vi "DataViewer_Optics.vi"() -> ()   [LabVIEW 2019]
uses:
  <vilib>/Utility/file.llb/Read Delimited Spreadsheet (DBL).vi
panel:
  in  "Tab Control":T1(tab)
  out "Spectrum":cluster{dbl[], "all rows":dbl[]}(graph)
  in  "Spectrum File":path
  in  "Calibration File":path
  in  "Spectrum":bool
  in  "Mask A":path
  out "Mask A Transmission":dbl[][](graph)
  in  "Transmission":bool
  out "Mask B Transmission":dbl[][](graph)
  in  "Mask B":path
  in  "Pixel to Plot":dbl
  in  "Transmission_Px":bool
  in  "Mask A":path
  in  "Mask B":path
  out "Mask A":dbl[](graph)
  out "Mask B":dbl[](graph)
  in  "Pixel":dbl
  in  "Phase":bool
  in  "Directory":path
  out "SLM Phase Mask A":cluster{"all rows":dbl[], "all rows":dbl[]}(graph)
  out "SLM Phase Mask B":cluster{"all rows":dbl[], "all rows":dbl[]}(graph)
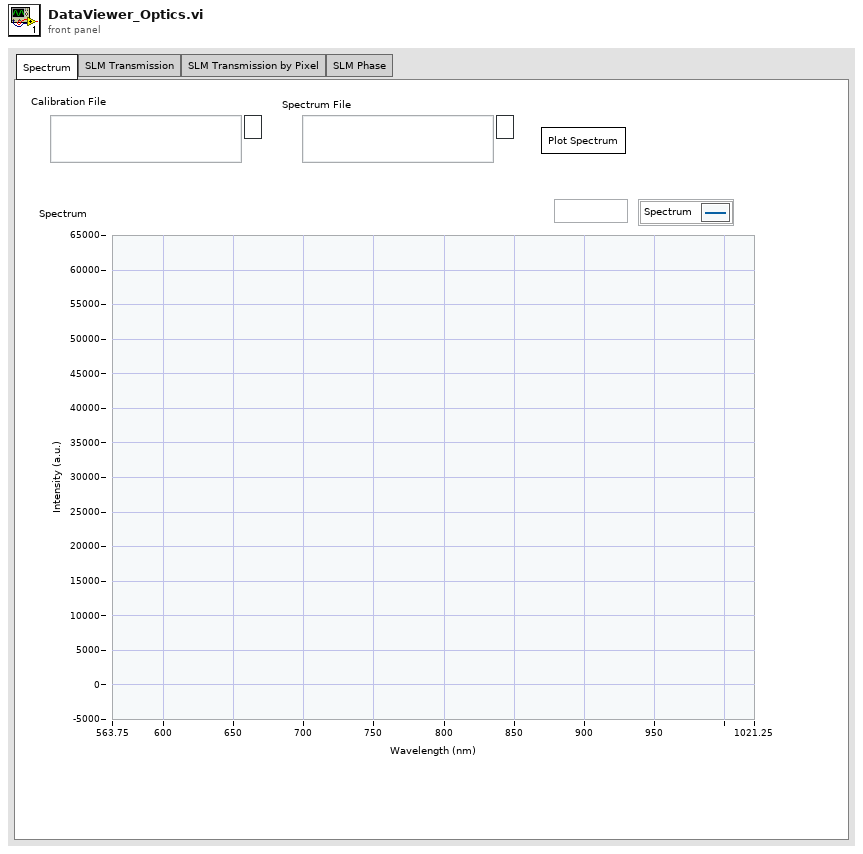
[diagram p1: front panel]
types:
  T1 = enum32{"Spectrum", "SLM Transmission", "SLM Transmission by Pixel", "SLM Phase"}
  T2 = enum32{"Invalid", "Standard", "Closed", "Hidden", "Minimized", "Maximized"}
  T3 = enum32{"invalid app kind", "Development System", "Run Time System", "Student Edition", "Embedded LabVIEW", "Evaluation", "Custom"}
  T4 = cluster{"Core":cluster{"Current VI Reference":refnum<vi>, "Close Panel on Exit?":bool}, "Your Boolean data":bool, "Your string data":string}
  T5 = cluster{"Current VI Reference":refnum<vi>, "Close Panel on Exit?":bool}
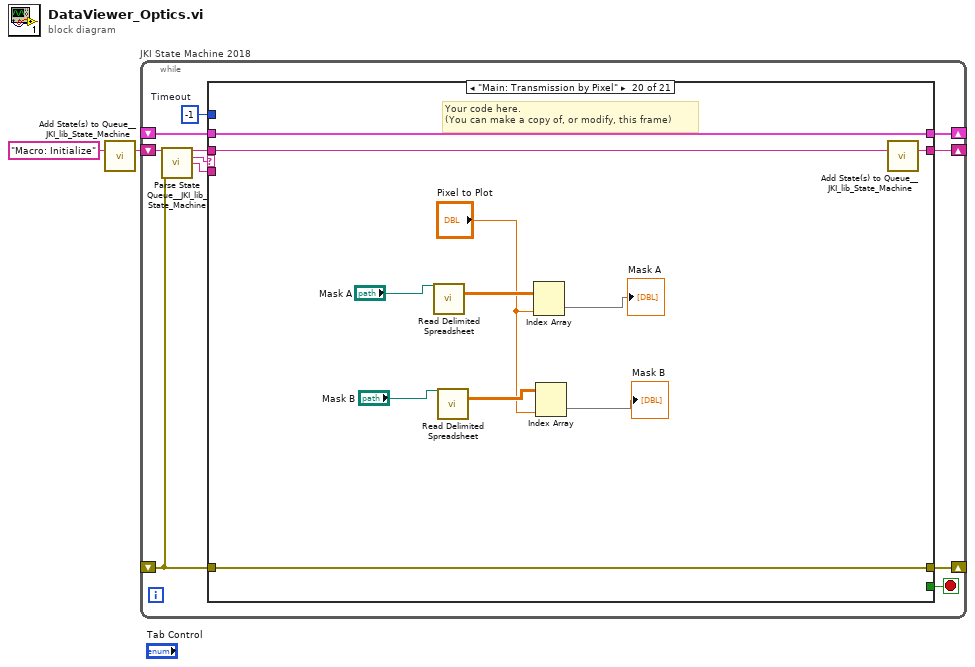
[diagram p0: block diagram]
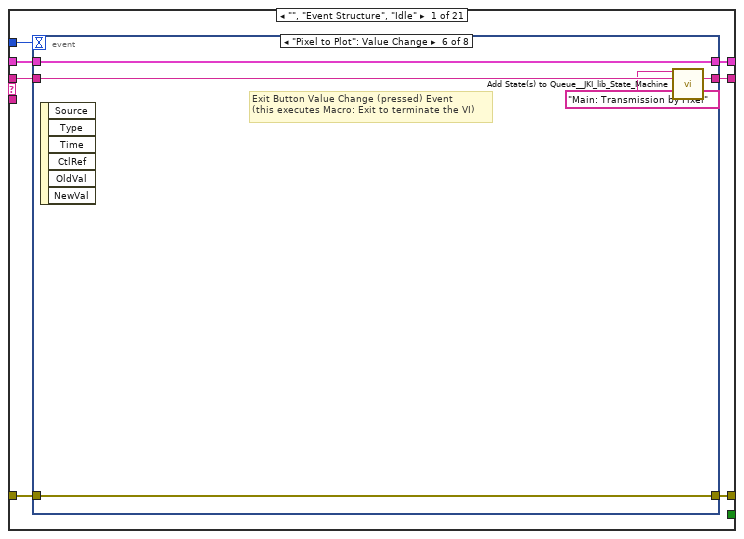
[diagram p2: hidden frame]
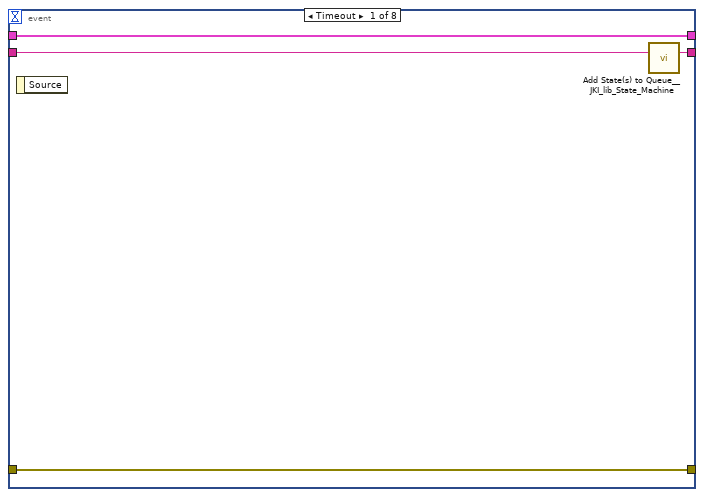
[diagram p3: hidden frame]
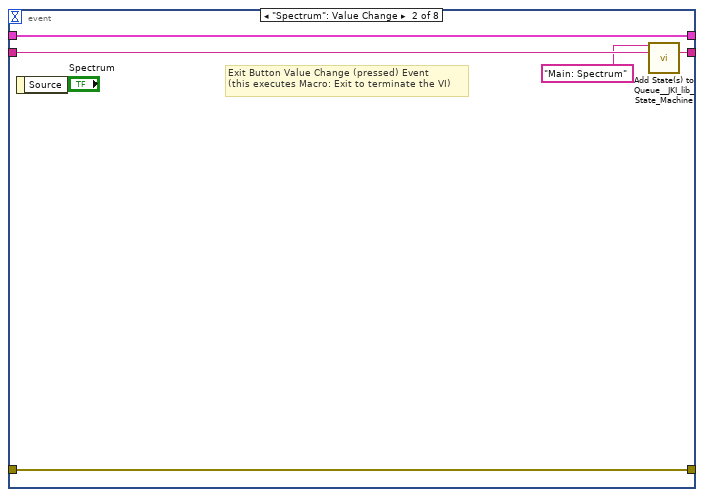
[diagram p4: hidden frame]
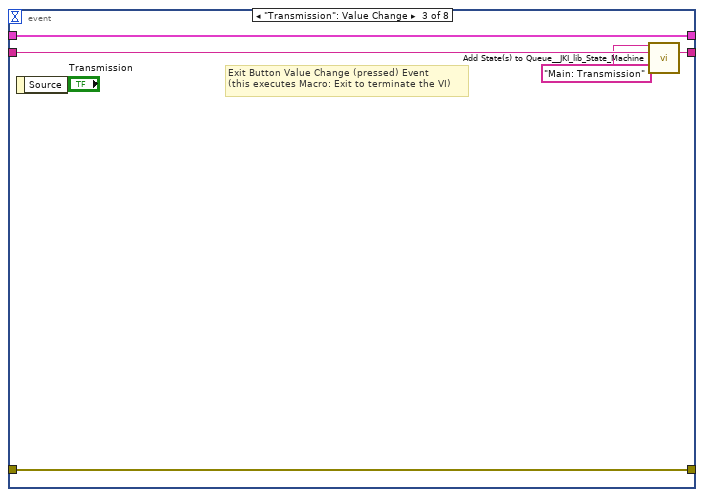
[diagram p5: hidden frame]
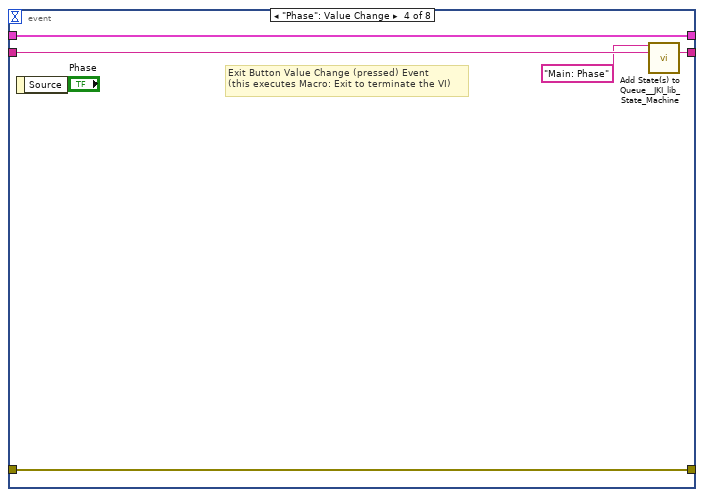
[diagram p6: hidden frame]
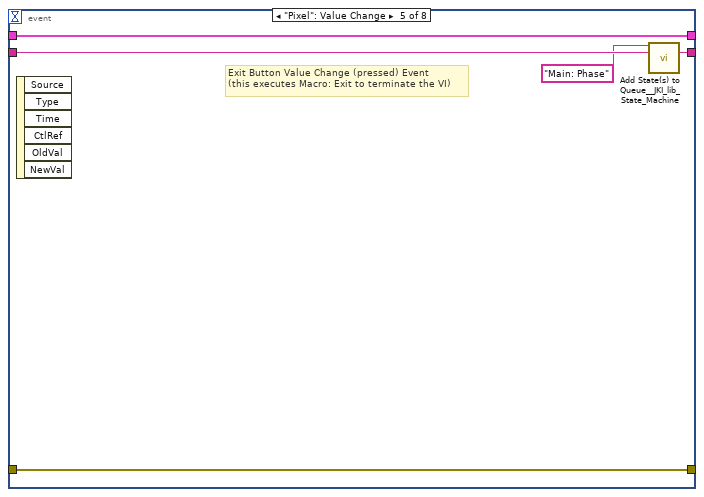
[diagram p7: hidden frame]
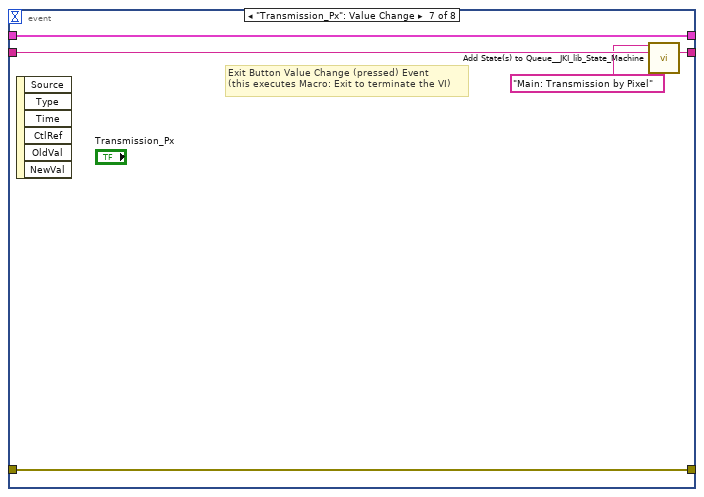
[diagram p8: hidden frame]
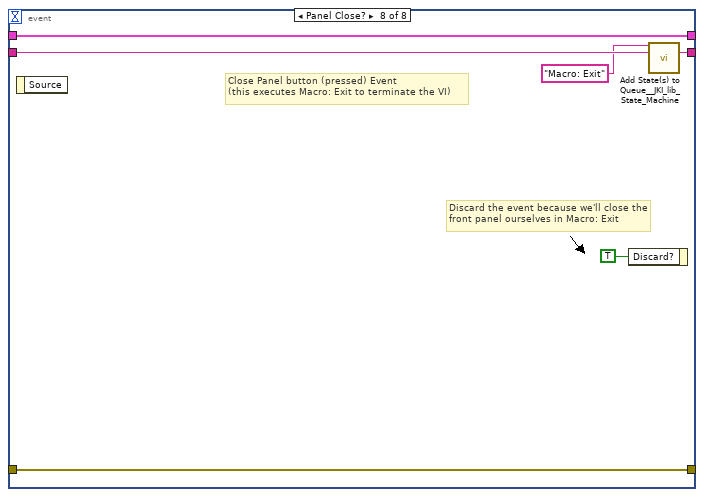
[diagram p9: hidden frame]
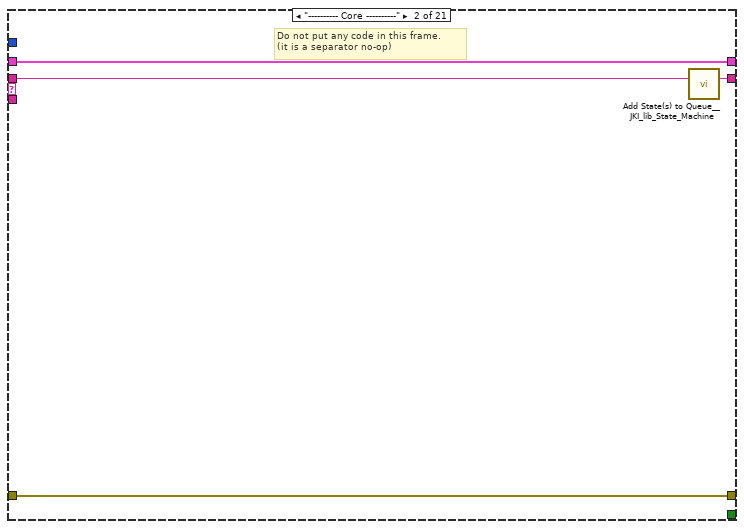
[diagram p10: hidden frame]
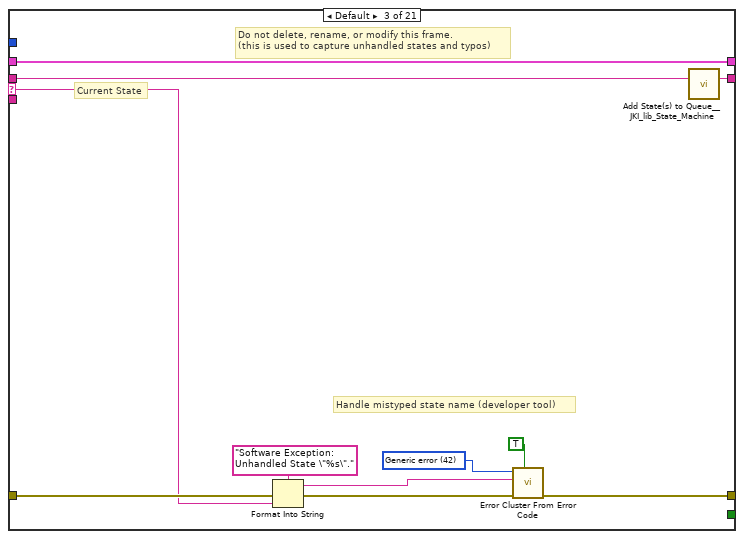
[diagram p11: hidden frame]
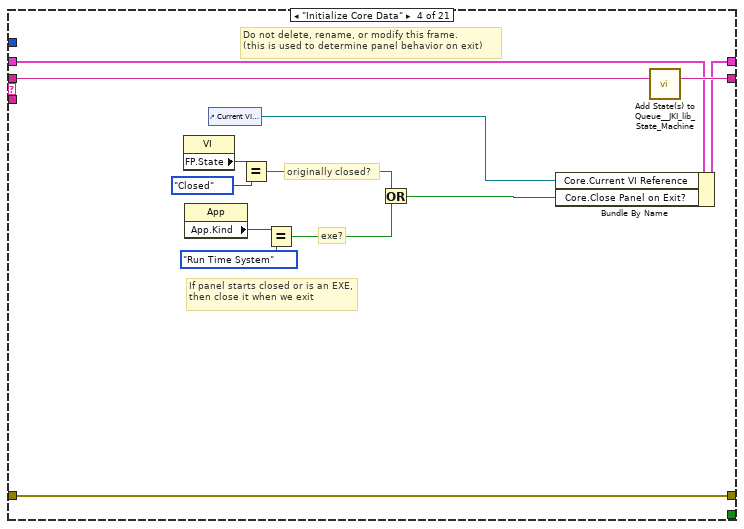
[diagram p12: hidden frame]
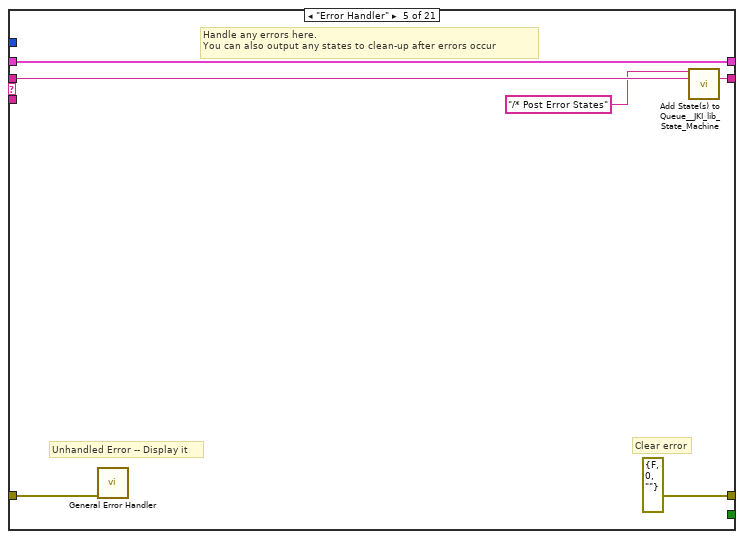
[diagram p13: hidden frame]
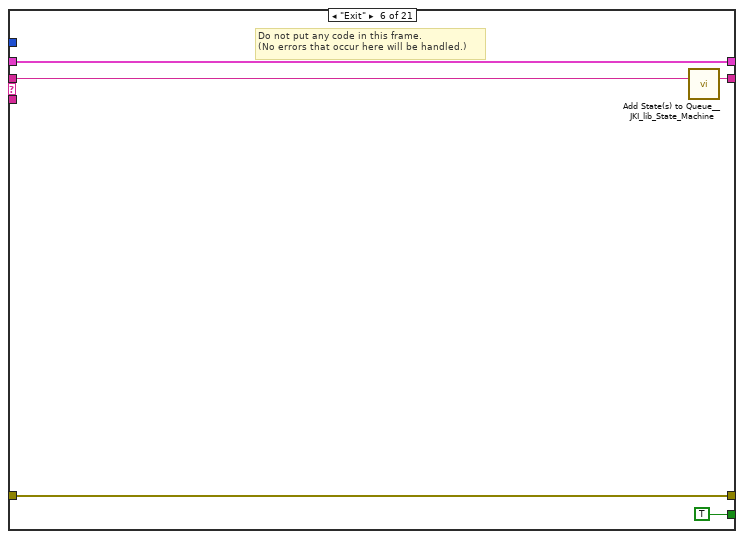
[diagram p14: hidden frame]
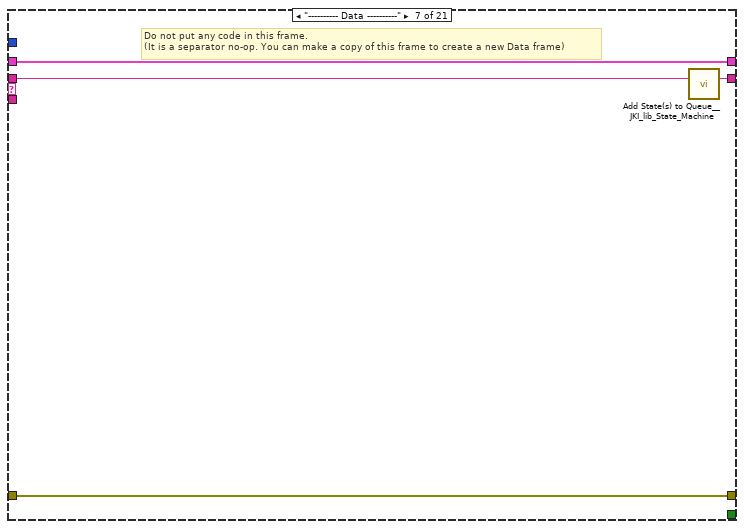
[diagram p15: hidden frame]
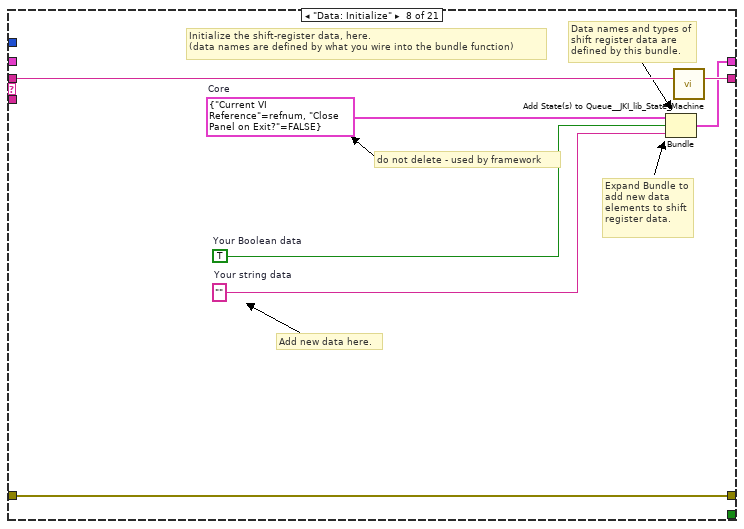
[diagram p16: hidden frame]
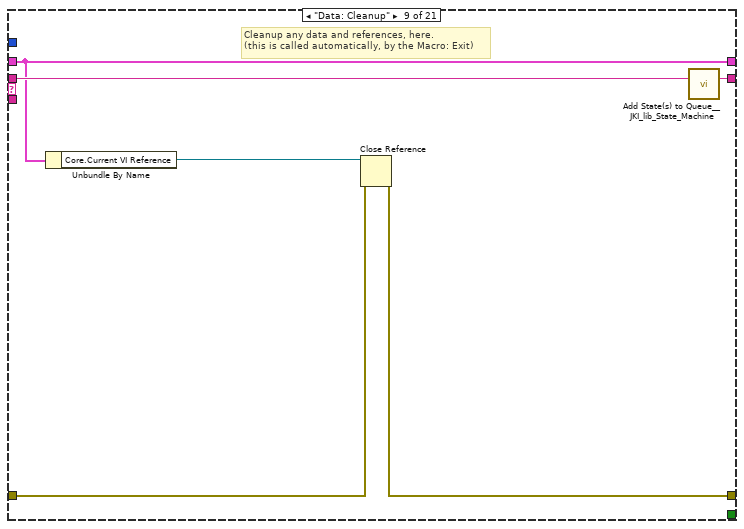
[diagram p17: hidden frame]
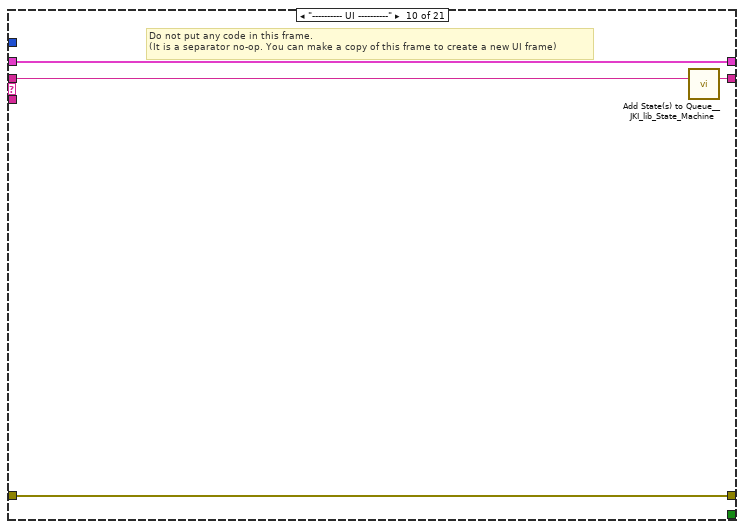
[diagram p18: hidden frame]
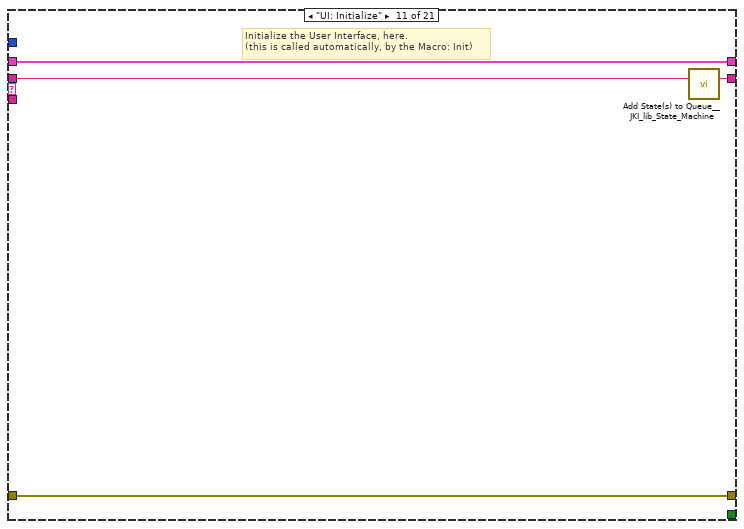
[diagram p19: hidden frame]
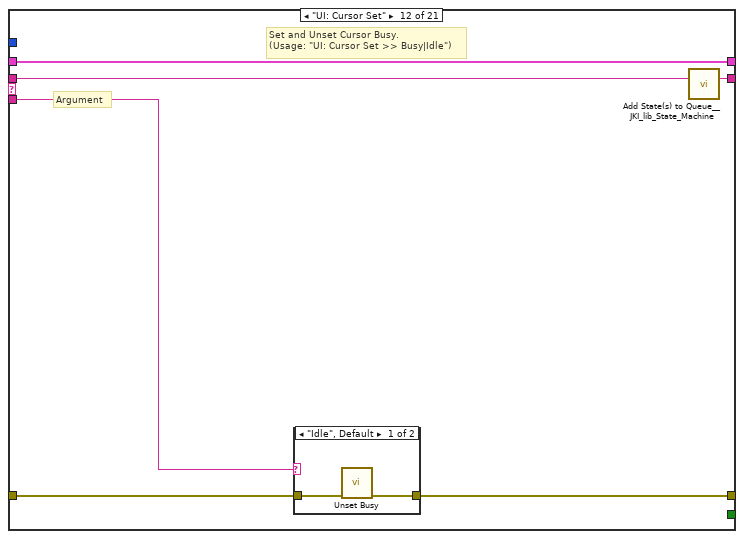
[diagram p20: hidden frame]
diagram:
  n1 = call <vilib>:"Add State(s) to Queue__JKI_lib_State_Machine.vi"("State(s) in (\"\")"="Macro: Initialize") -> ("States Out"=w2:string)  [unwired: 14 in]
  n2 = while "JKI State Machine 2018" {
    shift-right: [w6] -> _
    shift-left: _ -> [w5]
    shift-right: [w9] -> _
    shift-left: _ -> [w3]
    shift-right: [w8] -> _
    shift-left: w2 -> [w10]
    stop <- w7 stop-if-true
    w4 = -1  # Timeout
    n3 = call <vilib>:"Parse State Queue__JKI_lib_State_Machine.vi"("State Queue"=w10, "Error In (no error)"=w3) -> ("Remaining States"=w12:string, "Current State"=w13:string, "Arguments"=w11:string)  [unwired: 11 in]
    n4 = case shown="\"Main: Transmission by Pixel\"" w13 {
      selector: w13 -> [_ _ w65 _ _ _ _ _ _ _ _ _ _ _ _ _ _ _ _ _ _]
      tunnel: w12 -> [w20 w64 w69 w88 w94 w99 w103 w110 w116 w120 w124 w130 w141 w210 w215 w225 w229 w243 w251 w262 w288]
      tunnel: w11 -> [_ _ _ _ _ _ _ _ _ _ _ w125 w135 _ _ _ _ _ _ _ _]
      tunnel: w5 -> [w18 w61 w67 w81 w91 w97 w100 _ w111 w117 w122 w128 w137 w207 w212 w222 w226 w240 w248 w259 w286]
      tunnel: [w17 w62 w71 w85 errorcluster {"status"=FALSE, "code"=0, "source"=""} ("error out") w96 w101 w107 w112 w118 w121 w126 w138 w208 w213 w223 w227 w241 w249 w260 w263] -> w9
      tunnel: w3 -> [w16 w62 w70 w85 w90 w96 w101 w107 w113 w118 w121 w127 w139 w208 w213 w223 w227 w241 w249 w260 w265]
      tunnel: [w19 w63 w68 w87 w93 w98 w102 w109 w115 w119 w123 w129 w140 w209 w214 w224 w228 w242 w250 w261 w287] -> w8
      tunnel: [_ _ _ _ _ TRUE _ _ _ _ _ _ _ _ _ _ _ _ _ _ _] -> w7
      tunnel: [w15 w61 w67 w86 w91 w97 w100 w108 w111 w117 w122 w128 w137 w207 w212 w222 w226 w240 w248 w259 w286] -> w6
      tunnel: w4 -> [w14 _ _ _ _ _ _ _ _ _ _ _ _ _ _ _ _ _ _ _ _]
      frame "", "Event Structure", "Idle" {
        n5 = event shown="[5] \"Pixel to Plot\": Value Change" {
          selector: _ -> [_ _ _ _ _ _ _ _]
          dyn-events: _ -> [_ _ _ _ _ _ _ _]
          timeout: w14 -> [_ _ _ _ _ _ _ _]
          tunnel: w20 -> [w24 w29 w34 w39 w44 w49 w54 w60]
          tunnel: [w23 w28 w33 w38 w43 w48 w53 w59] -> w19
          tunnel: w18 -> [w21 w26 w31 w36 w41 w46 w51 w57]
          tunnel: [w22 w27 w32 w37 w42 w47 w52 w58] -> w17
          tunnel: w16 -> [w22 w27 w32 w37 w42 w47 w52 w58]
          tunnel: [w21 w26 w31 w36 w41 w46 w51 w57] -> w15
          event Timeout {
            n6 = event-data() -> ()  [unwired: 1 in, 1 out]
            n7 = call <vilib>:"Add State(s) to Queue__JKI_lib_State_Machine.vi"("State(s) in (\"\")"=w24) -> ("States Out"=w23:string)  [unwired: 14 in]
          }
          event "Spectrum": Value Change {
            # "Exit Button Value Change (pressed) Event\n(this executes Macro: Exit to terminate the VI)"
            n8 = event-data() -> ()  [unwired: 1 in, 1 out]
            n9 = call <vilib>:"Add State(s) to Queue__JKI_lib_State_Machine.vi"("State(s) in Front (\"\")"="Main: Spectrum", "State(s) in (\"\")"=w29) -> ("States Out"=w28:string)  [unwired: 13 in]
          }
          event "Transmission": Value Change {
            # "Exit Button Value Change (pressed) Event\n(this executes Macro: Exit to terminate the VI)"
            n10 = event-data() -> ()  [unwired: 1 in, 1 out]
            n11 = call <vilib>:"Add State(s) to Queue__JKI_lib_State_Machine.vi"("State(s) in Front (\"\")"="Main: Transmission", "State(s) in (\"\")"=w34) -> ("States Out"=w33:string)  [unwired: 13 in]
          }
          event "Phase": Value Change {
            # "Exit Button Value Change (pressed) Event\n(this executes Macro: Exit to terminate the VI)"
            n12 = event-data() -> ()  [unwired: 1 in, 1 out]
            n13 = call <vilib>:"Add State(s) to Queue__JKI_lib_State_Machine.vi"("State(s) in Front (\"\")"="Main: Phase", "State(s) in (\"\")"=w39) -> ("States Out"=w38:string)  [unwired: 13 in]
          }
          event "Pixel": Value Change {
            # "Exit Button Value Change (pressed) Event\n(this executes Macro: Exit to terminate the VI)"
            n14 = event-data() -> ()  [unwired: 1 in, 6 out]
            n15 = call <vilib>:"Add State(s) to Queue__JKI_lib_State_Machine.vi"("State(s) in Front (\"\")"="Main: Phase", "State(s) in (\"\")"=w44) -> ("States Out"=w43:string)  [unwired: 13 in]
          }
          event "Pixel to Plot": Value Change {
            # "Exit Button Value Change (pressed) Event\n(this executes Macro: Exit to terminate the VI)"
            n16 = event-data() -> ()  [unwired: 1 in, 6 out]
            n17 = call <vilib>:"Add State(s) to Queue__JKI_lib_State_Machine.vi"("State(s) in Front (\"\")"="Main: Transmission by Pixel", "State(s) in (\"\")"=w49) -> ("States Out"=w48:string)  [unwired: 13 in]
          }
          event "Transmission_Px": Value Change {
            # "Exit Button Value Change (pressed) Event\n(this executes Macro: Exit to terminate the VI)"
            n18 = event-data() -> ()  [unwired: 1 in, 6 out]
            n19 = call <vilib>:"Add State(s) to Queue__JKI_lib_State_Machine.vi"("State(s) in Front (\"\")"="Main: Transmission by Pixel", "State(s) in (\"\")"=w54) -> ("States Out"=w53:string)  [unwired: 13 in]
          }
          event Panel Close? {
            # "Discard the event because we'll close the front panel ourselves in Macro: Exit"
            # "Close Panel button (pressed) Event\n(this executes Macro: Exit to terminate the VI)"
            n20 = event-data() -> ()  [unwired: 1 in, 1 out]
            n21 = event-data("Discard?"=TRUE) -> ()  [unwired: 1 in, 1 out]
            n22 = call <vilib>:"Add State(s) to Queue__JKI_lib_State_Machine.vi"("State(s) in Front (\"\")"="Macro: Exit", "State(s) in (\"\")"=w60) -> ("States Out"=w59:string)  [unwired: 13 in]
          }
        }
      }
      frame "---------- Core ----------" {
        # "Do not put any code in this frame.\n(it is a separator no-op)"
        n23 = call <vilib>:"Add State(s) to Queue__JKI_lib_State_Machine.vi"("State(s) in (\"\")"=w64) -> ("States Out"=w63:string)  [unwired: 14 in]
      }
      frame Default {
        w74 = 42 items=["No error", "Argument error", "Memory is full", "Out of zone", "End of file", "File already open", "Generic file I/O error", "File not found", "File permission error", "Disk is full", "Duplicate path", "Too many files open", "System feature not enabled", "Resource file not found", "Cannot add resource", "Resource not found", "Image not found", "Image memory error", "Pen does not exist", "Config type invalid", "Config token not found", "Config parse error", "Config memory error", "Bad external code format", "Bad external code offset", "External code not present", "Null window", "Destroy window error", "Null menu", "Print aborted", "Bad print record", "Print driver error", "Windows error during printing", "Memory error during printing", "Print dialog error", "Generic print error", "Invalid device refnum", "Device not found", "Device parameter error", "Device unit error", "Cannot open device", "Device call aborted", "Generic error", "Cancelled by user", "Object ID too low", "Object ID too high", "Object not in heap", "Unknown heap", "Unknown object (invalid DefProc)", "Unknown object (DefProc not in table)", "Message out of range", "Invalid (null) method", "Unknown message", "Manager call not supported", "Bad address", "Network operation in progress", "Network operation timed out", "Connection is busy", "Network attribute not supported", "Network error", "Address in use", "System out of memory", "Connection aborted", "Connection refused", "Not connected", "Already connected", "Connection closed", "Initialization error (interapplication manager)", "Bad occurrence", "Wait on unbound occurrence handler", "Occurrence queue overflow", "Datalog type conflict", "Unused", "Unrecognized type (interapplication manager)", "Memory corrupt", "Failed to make temporary DLL", "Old CIN version", "Drag socket not found", "Failed to load drop-object", "Failed to register OLE object", "Failed to release OLE object", "Format specifier type mismatch", "Unknown format specifier", "Too few format specifiers", "Too many format specifiers", "Scan failed", "Newer CIN version", "Error converting to variant", "Runtime menu error", "Password tampered", "Variant attribute not found", "Incompatible variant data type", "Event data is not available", "Event Store is not present", "Occurrence is not found", "Event Queue is not created", "Event info is not available", "Refnum passed is NULL", "Error retrieving Class GUID", "Error retrieving CoClass GUID", "Error retrieving TypeLib GUID.", "Bad built application magic bytes.", "Specific driver is different from the specific driver associated with the Logical Name.", "There is no session opened to the class driver.", "Max Error", "MAX - Error with config objects", "MAX - Error loading configuration", "MAX - Group not supported"]
        # "Current State"
        # "Do not delete, rename, or modify this frame.\n(this is used to capture unhandled states and typos)"
        # "Handle mistyped state name (developer tool)"
        n24 = Format Into String(format string="Software Exception: Unhandled State \"%s\"." ("message"), error in=w70, w65) -> (resulting string=w73:string, error out=w72:errorcluster)  [unwired: 1 in]
        n25 = call <vilib>:"Error Cluster From Error Code.vi"("show call chain? (False)"=TRUE, "error in (no error)"=w72, "error message (\"\")"=w73, "error code (0)"=w74) -> ("error out"=w71:errorcluster)  [unwired: 5 in]
        n26 = call <vilib>:"Add State(s) to Queue__JKI_lib_State_Machine.vi"("State(s) in (\"\")"=w69) -> ("States Out"=w68:string)  [unwired: 14 in]
      }
      frame "Initialize Core Data" {
        # "Do not delete, rename, or modify this frame.\n(this is used to determine panel behavior on exit)"
        # "originally closed?"
        # "exe?"
        # "If panel starts closed or is an EXE, then close it when we exit"
        n27 = property class="VI"() -> ("FP.State"=w78:T2)  [unwired: 2 in, 2 out]
        n28 = property class="App"() -> ("App.Kind"=w84:T3)  [unwired: 2 in, 2 out]
        n29 = control-ref of="Current VI Reference"() -> (w79:refnum<vi>)
        n30 = Equal?(x=w78, y=T2."Closed" ("Front Panel Window:State")) -> (x = y?=w76:bool)
        n31 = Equal?(x=w84, y=T3."Run Time System" ("Application:Kind")) -> (x = y?=w82:bool)
        n32 = Or(x=w76, y=w82) -> (x .or. y?=w80:bool)
        n33 = Bundle By Name(cluster=w81, "Core.Current VI Reference"=w79, "Core.Close Panel on Exit?"=w80) -> (w86:T4)
        n34 = call <vilib>:"Add State(s) to Queue__JKI_lib_State_Machine.vi"("State(s) in (\"\")"=w88) -> ("States Out"=w87:string)  [unwired: 14 in]
      }
      frame "Error Handler" {
        # "Unhandled Error -- Display it"
        # "Handle any errors here.\nYou can also output any states to clean-up after errors occur"
        # "Clear error"
        n35 = call <vilib>:"General Error Handler.vi"("error in (no error)"=w90) -> ()  [unwired: 10 in, 5 out]
        n36 = call <vilib>:"Add State(s) to Queue__JKI_lib_State_Machine.vi"("State(s) in Front (\"\")"="/* Post Error States", "State(s) in (\"\")"=w94) -> ("States Out"=w93:string)  [unwired: 13 in]
      }
      frame "Exit" {
        # "Do not put any code in this frame.\n(No errors that occur here will be handled.)"
        n37 = call <vilib>:"Add State(s) to Queue__JKI_lib_State_Machine.vi"("State(s) in (\"\")"=w99) -> ("States Out"=w98:string)  [unwired: 14 in]
      }
      frame "---------- Data ----------" {
        # "Do not put any code in this frame.\n(It is a separator no-op. You can make a copy of this frame to create a new Data frame)"
        n38 = call <vilib>:"Add State(s) to Queue__JKI_lib_State_Machine.vi"("State(s) in (\"\")"=w103) -> ("States Out"=w102:string)  [unwired: 14 in]
      }
      frame "Data: Initialize" {
        w104 = T5 {"Current VI Reference"=refnum, "Close Panel on Exit?"=FALSE}  # Core
        w106 = TRUE  # Your Boolean data
        w105 = ""  # Your string data
        # "do not delete - used by framework"
        # "Expand Bundle to add new data elements to shift register data."
        # "Add new data here."
        # "Data names and types of shift register data are defined by this bundle."
        # "Initialize the shift-register data, here.\n(data names are defined by what you wire into the bundle function)"
        n39 = Bundle("Core"=w104, "Your Boolean data"=w106, "Your string data"=w105) -> (w108:T4)  [unwired: 1 in]
        n40 = call <vilib>:"Add State(s) to Queue__JKI_lib_State_Machine.vi"("State(s) in (\"\")"=w110) -> ("States Out"=w109:string)  [unwired: 14 in]
      }
      frame "Data: Cleanup" {
        # "Cleanup any data and references, here.\n(this is called automatically, by the Macro: Exit)"
        n41 = Unbundle By Name(w111) -> ("Core.Current VI Reference"=w114:refnum<vi>)
        n42 = Close Reference(reference=w114, error in (no error)=w113) -> (error out=w112:errorcluster)
        n43 = call <vilib>:"Add State(s) to Queue__JKI_lib_State_Machine.vi"("State(s) in (\"\")"=w116) -> ("States Out"=w115:string)  [unwired: 14 in]
      }
      frame "---------- UI ----------" {
        # "Do not put any code in this frame.\n(It is a separator no-op. You can make a copy of this frame to create a new UI frame)"
        n44 = call <vilib>:"Add State(s) to Queue__JKI_lib_State_Machine.vi"("State(s) in (\"\")"=w120) -> ("States Out"=w119:string)  [unwired: 14 in]
      }
      frame "UI: Initialize" {
        # "Initialize the User Interface, here.\n(this is called automatically, by the Macro: Init)"
        n45 = call <vilib>:"Add State(s) to Queue__JKI_lib_State_Machine.vi"("State(s) in (\"\")"=w124) -> ("States Out"=w123:string)  [unwired: 14 in]
      }
      frame "UI: Cursor Set" {
        # "Argument"
        # "Set and Unset Cursor Busy.\n(Usage: \"UI: Cursor Set >> Busy|Idle\")"
        n46 = case shown="\"Idle\", Default" w125 {
          tunnel: w127 -> [w132 w134]
          tunnel: [w131 w133] -> w126
          frame "Idle", Default {
            n47 = call <vilib>:"Unset Busy.vi"("error in (no error)"=w132) -> ("error out"=w131:errorcluster)  [unwired: 10 in]
          }
          frame "Busy" {
            n48 = call <vilib>:"Set Busy.vi"("error in (no error)"=w134) -> ("error out"=w133:errorcluster)  [unwired: 9 in, 1 out]
          }
        }
        n49 = call <vilib>:"Add State(s) to Queue__JKI_lib_State_Machine.vi"("State(s) in (\"\")"=w130) -> ("States Out"=w129:string)  [unwired: 14 in]
      }
      frame "UI: Front Panel State" {
        # "Argument"
        # "Set Front Panel Open or Closed\n(Usage: \"UI: Front Panel State >> Open|Close\")"
        n50 = Unbundle By Name(w137) -> ("Core.Current VI Reference"=w136:refnum<vi>)
        n51 = case shown="\"Minimize\", \"Minimized\"" w135 {
          tunnel: w139 -> [w147 w162 w173 w186 w199]
          tunnel: [w149 w163 w175 w188 w201] -> w138
          tunnel: w136 -> [w148 w160 w174 w187 w200]
          frame "Open", "Standard", Default {
            w142 = T2."Standard" ("State")
            n52 = property class="VI"(reference=w148, error in=w147) -> (reference out=w145:refnum<vi>, error out=w146:errorcluster, "FP.State"=w144:T2)
            n53 = Not Equal?(x=w144, y=w142) -> (x != y?=w143:bool)
            n54 = case shown="True" w143 {
              tunnel: [w153 w155] -> w149
              tunnel: w146 -> [w152 w155]
              tunnel: w145 -> [w151 _]
              tunnel: w142 -> [w150 _]
              frame True {
                n55 = invoke class="VI" method="FP.Open"(reference=w151, error in=w152, "Activate"=TRUE, "State"=w150) -> (error out=w153:errorcluster)  [unwired: 1 in, 4 out]
              }
              frame False {
              }
            }
          }
          frame "Close", "Closed" {
            n56 = property class="VI"(reference=w160, error in=w162) -> (reference out=w159:refnum<vi>, error out=w161:errorcluster, "FP.State"=w157:T2)
            n57 = Not Equal?(x=w157, y=T2."Closed" ("Front Panel Window:State")) -> (x != y?=w156:bool)
            n58 = case shown="True" w156 {
              tunnel: [w164 w167] -> w163
              tunnel: w161 -> [w164 w166]
              tunnel: w159 -> [_ w165]
              frame False {
              }
              frame True {
                n59 = invoke class="VI" method="FP.Close"(reference=w165, error in=w166) -> (error out=w167:errorcluster)  [unwired: 1 in, 2 out]
              }
            }
          }
          frame "Hidden", "Hide" {
            w168 = T2."Hidden" ("State")
            n60 = property class="VI"(reference=w174, error in=w173) -> (reference out=w171:refnum<vi>, error out=w172:errorcluster, "FP.State"=w170:T2)
            n61 = Not Equal?(x=w170, y=w168) -> (x != y?=w169:bool)
            n62 = case shown="True" w169 {
              tunnel: [w179 w180] -> w175
              tunnel: w172 -> [w178 w180]
              tunnel: w171 -> [w177 _]
              tunnel: w168 -> [w176 _]
              frame True {
                n63 = invoke class="VI" method="FP.Open"(reference=w177, error in=w178, "State"=w176) -> (error out=w179:errorcluster)  [unwired: 2 in, 4 out]
              }
              frame False {
              }
            }
          }
          frame "Minimize", "Minimized" {
            w181 = T2."Minimized" ("State")
            n64 = property class="VI"(reference=w187, error in=w186) -> (reference out=w184:refnum<vi>, error out=w185:errorcluster, "FP.State"=w183:T2)
            n65 = Not Equal?(x=w183, y=w181) -> (x != y?=w182:bool)
            n66 = case shown="True" w182 {
              tunnel: [w192 w193] -> w188
              tunnel: w185 -> [w191 w193]
              tunnel: w184 -> [w190 _]
              tunnel: w181 -> [w189 _]
              frame True {
                n67 = invoke class="VI" method="FP.Open"(reference=w190, error in=w191, "State"=w189) -> (error out=w192:errorcluster)  [unwired: 2 in, 4 out]
              }
              frame False {
              }
            }
          }
          frame "Maximize", "Maximized" {
            w194 = T2."Maximized" ("State")
            n68 = property class="VI"(reference=w200, error in=w199) -> (reference out=w197:refnum<vi>, error out=w198:errorcluster, "FP.State"=w196:T2)
            n69 = Not Equal?(x=w196, y=w194) -> (x != y?=w195:bool)
            n70 = case shown="True" w195 {
              tunnel: [w205 w206] -> w201
              tunnel: w198 -> [w204 w206]
              tunnel: w197 -> [w203 _]
              tunnel: w194 -> [w202 _]
              frame True {
                n71 = invoke class="VI" method="FP.Open"(reference=w203, error in=w204, "State"=w202) -> (error out=w205:errorcluster)  [unwired: 2 in, 4 out]
              }
              frame False {
              }
            }
          }
        }
        n72 = call <vilib>:"Add State(s) to Queue__JKI_lib_State_Machine.vi"("State(s) in (\"\")"=w141) -> ("States Out"=w140:string)  [unwired: 14 in]
      }
      frame "---------- Macro ----------" {
        # "Do not put any code in this frame.\n(It is a separator no-op. You can make a copy of this frame to create a new Macro frame)"
        n73 = call <vilib>:"Add State(s) to Queue__JKI_lib_State_Machine.vi"("State(s) in (\"\")"=w210) -> ("States Out"=w209:string)  [unwired: 14 in]
      }
      frame "Macro: Initialize" {
        w211 = "Data: Initialize\nInitialize Core Data\nUI: Initialize\nUI: Front Panel State >> Open"  # Data: Initialize Initialize Core Data UI: Initialize UI: Front Panel State >> Open
        # "Initialization Macro\n(This is called once, when the VI starts)"
        n74 = call <vilib>:"Add State(s) to Queue__JKI_lib_State_Machine.vi"("State(s) in Front (\"\")"=w211, "State(s) in (\"\")"=w215) -> ("States Out"=w214:string)  [unwired: 13 in]
      }
      frame "Macro: Exit" {
        # "Exit Macro\n(This is called once, when the VI exits)"
        n75 = Unbundle By Name(w222) -> ("Core.Close Panel on Exit?"=w221:bool)
        n76 = Select(t="UI: Front Panel State >> Close", s=w221, f="") -> (s? t:f=w218:string)
        n77 = call <vilib>:"Add State(s) to Queue__JKI_lib_State_Machine.vi"("State(s) in (\"\")"=w218, "State(s) at Back (\"\")"="Data: Cleanup\nExit") -> ("States Out"=w216:string)  [unwired: 13 in]
        n78 = call <vilib>:"Add State(s) to Queue__JKI_lib_State_Machine.vi"("State(s) in Front (\"\")"=w216, "State(s) in (\"\")"=w225) -> ("States Out"=w224:string)  [unwired: 13 in]
      }
      frame "---------- Main ----------" {
        # "Template Separator\n(You can make a copy of, or modify, this frame)"
        n79 = call <vilib>:"Add State(s) to Queue__JKI_lib_State_Machine.vi"("State(s) in (\"\")"=w229) -> ("States Out"=w228:string)  [unwired: 14 in]
      }
      frame "Main: Spectrum" {
        # "Your code here.\n(You can make a copy of, or modify, this frame)"
        n80 = call-poly <vilib>:"Read Delimited Spreadsheet.vi"("file path (dialog if empty)"="Calibration File") -> ("all rows"=w239:dbl[][])  [unwired: 9 in, 5 out]
        n81 = call-poly <vilib>:"Read Delimited Spreadsheet.vi"("file path (dialog if empty)"="Spectrum File") -> ("all rows"=w235:dbl[][])  [unwired: 9 in, 5 out]
        n82 = Index Array(array=w239, index (col)=0) -> (element=w238:dbl[])  [unwired: 1 in]
        n83 = Reverse 1D Array(array=w238) -> (reversed array=w230:dbl[])
        n84 = Index Array(array=w235, index (row)=0 ("disabled index (col)")) -> (element=w234:dbl[])  [unwired: 1 in]
        n85 = Bundle(w230, "all rows"=w234) -> (→"Spectrum":cluster{dbl[], "all rows":dbl[]})  [unwired: 1 in]
        n86 = call <vilib>:"Add State(s) to Queue__JKI_lib_State_Machine.vi"("State(s) in (\"\")"=w243) -> ("States Out"=w242:string)  [unwired: 14 in]
      }
      frame "Main: Transmission" {
        # "Your code here.\n(You can make a copy of, or modify, this frame)"
        n87 = call-poly <vilib>:"Read Delimited Spreadsheet.vi"("file path (dialog if empty)"="Mask A") -> ("all rows"=→"Mask A Transmission":dbl[][])  [unwired: 9 in, 5 out]
        n88 = call-poly <vilib>:"Read Delimited Spreadsheet.vi"("file path (dialog if empty)"="Mask B") -> ("all rows"=→"Mask B Transmission":dbl[][])  [unwired: 9 in, 5 out]
        n89 = call <vilib>:"Add State(s) to Queue__JKI_lib_State_Machine.vi"("State(s) in (\"\")"=w251) -> ("States Out"=w250:string)  [unwired: 14 in]
      }
      frame "Main: Transmission by Pixel" {
        # "Your code here.\n(You can make a copy of, or modify, this frame)"
        n90 = call-poly <vilib>:"Read Delimited Spreadsheet.vi"("file path (dialog if empty)"="Mask A") -> ("all rows"=w256:dbl[][])  [unwired: 9 in, 5 out]
        n91 = call-poly <vilib>:"Read Delimited Spreadsheet.vi"("file path (dialog if empty)"="Mask B") -> ("all rows"=w255:dbl[][])  [unwired: 9 in, 5 out]
        n92 = Index Array(array=w256, index (col)="Pixel to Plot") -> (element=→"Mask A":dbl[])  [unwired: 1 in]
        n93 = Index Array(array=w255, index (col)="Pixel to Plot") -> (element=→"Mask B":dbl[])  [unwired: 1 in]
        n94 = call <vilib>:"Add State(s) to Queue__JKI_lib_State_Machine.vi"("State(s) in (\"\")"=w262) -> ("States Out"=w261:string)  [unwired: 14 in]
      }
      frame "Main: Phase" {
        # "Your code here.\n(You can make a copy of, or modify, this frame)"
        n95 = Number To Decimal String(number="Pixel") -> (decimal integer string=w268:string)  [unwired: 1 in]
        n96 = Path To String(path="Directory") -> (string=w270:string)
        n97 = Concatenate Strings(w270, "\\Mask B\\Mask_B_phase_pixel_" ("string"), w268) -> (w267:string)
        n98 = Concatenate Strings(w270, "\\Mask A\\Mask_A_phase_pixel_" ("string"), w268) -> (w272:string)
        n99 = String To Path(string=w267) -> (path=w266:path)
        n100 = String To Path(string=w272) -> (path=w271:path)
        n101 = call-poly <vilib>:"Read Delimited Spreadsheet.vi"("file path (dialog if empty)"=w271, "error in (no error)"=w265) -> ("all rows"=w285:dbl[][], "error out"=w264:errorcluster)  [unwired: 8 in, 4 out]
        n102 = call-poly <vilib>:"Read Delimited Spreadsheet.vi"("file path (dialog if empty)"=w266, "error in (no error)"=w264) -> ("all rows"=w280:dbl[][], "error out"=w263:errorcluster)  [unwired: 8 in, 4 out]
        n103 = Index Array(array=w280, index (col) #1=0 ("disabled index (col)")) -> (element #1=w278:dbl[], element #2=w277:dbl[])  [unwired: 3 in]
        n104 = Index Array(array=w285, index (col) #1=0 ("disabled index (col)")) -> (element #1=w283:dbl[], element #2=w282:dbl[])  [unwired: 3 in]
        n105 = Bundle("all rows"=w278, "all rows"=w277) -> (→"SLM Phase Mask B":cluster{"all rows":dbl[], "all rows":dbl[]})  [unwired: 1 in]
        n106 = Bundle("all rows"=w283, "all rows"=w282) -> (→"SLM Phase Mask A":cluster{"all rows":dbl[], "all rows":dbl[]})  [unwired: 1 in]
        n107 = call <vilib>:"Add State(s) to Queue__JKI_lib_State_Machine.vi"("State(s) in (\"\")"=w288) -> ("States Out"=w287:string)  [unwired: 14 in]
      }
    }
  }
